vi "receive.vi"(0 "object in":refnum<class "tcp_work.lvclass">, 5 "error in (no error)":errorcluster) -> (14 "object out":refnum<class "tcp_work.lvclass">, 15 "读取缓冲区":string, 16 "返回数":u32, 19 "error out":errorcluster)   [LabVIEW 2016, in "tcp_work.lvclass"]
uses:
  tcp_work.lvclass
  tcp_work.lvclass/tcp_work.ctl
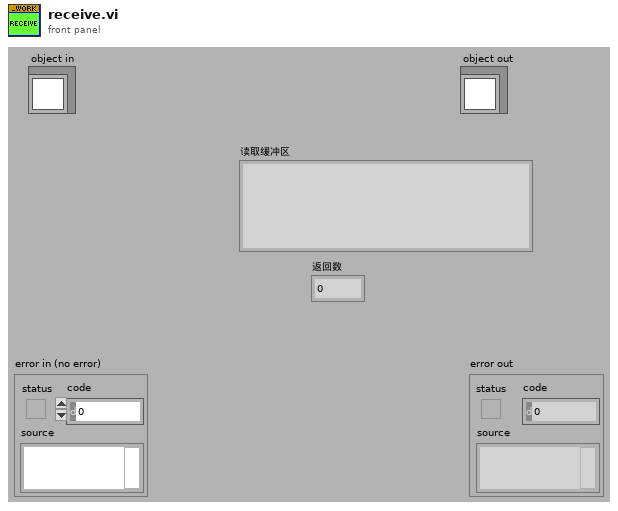
[diagram p1: front panel]
types:
  T1 = enum16{"Standard", "Buffered", "CRLF", "Immediate"}
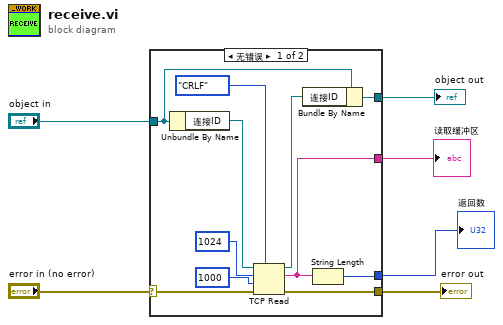
[diagram p0: block diagram]
diagram:
  n1 = case shown="无错误" "error in (no error)" {
    selector: "error in (no error)" -> [w11 w19]
    tunnel: [w10 w19] -> w5
    tunnel: [w16 w18] -> w3
    tunnel: "object in" -> [w17 w18]
    tunnel: [w8 _] -> w2
    tunnel: [w7 _] -> w1
    frame No Error {
      n2 = Unbundle By Name(w17) -> ("连接ID"=w12:refnum<k5>)
      n3 = TCP Read(connection ID=w12, bytes to read=1024 ("读取的字节"), error in (no error)=w11, 7:T1."CRLF" ("模式（标准）"), 9:1000 ("超时毫秒(25000)")) -> (connection ID out=w9:refnum<k5>, data out=w8:string, error out=w10:errorcluster)
      n4 = Bundle By Name(cluster=w17, "连接ID"=w9) -> (w16:refnum<class "tcp_work.lvclass">)
      n5 = String Length(string=w8) -> (length=w7:i32)
    }
    frame Error {
    }
  }
  "error out" <- w5
  "object out" <- w3
  "读取缓冲区" <- w2
  "返回数" <- w1
